vi "CODMn启动命令 (子VI).vi"(10 "CODMn量程切换":enum32{"H", "L", "AUTO"}(ring)=enum."AUTO", 11 "启动测量模式":T1) -> ()   [LabVIEW 2016, in "斯坦道CODMn.lvlib"]
uses:
  <vilib>/Plasmionique/MB Master/MB_Master_Serial/MB_Master_Serial.lvclass
  C:/Program Files (x86)/National Instruments/LabVIEW 2016/vi.lib/Plasmionique/MB Master/MB_Master/MB_Master.lvclass
  <vilib>/Plasmionique/MB Master/MB Master.lvlib
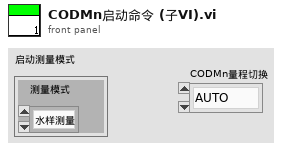
[diagram p1: front panel]
types:
  T1 = cluster{"测量模式":enum16{"水样测量", "标样核查", "零点核查", "跨度核查", "空白测试", "加标回收", "平行样", "校零", "校标"}}
  T2 = cluster{"baud rate (bps)":u32, "stop bits":u16, "parity":u16, "flow control":u16, "timeout":u32, "retries":i32}
  T3 = enum16{"水样测量", "标样核查", "零点核查", "跨度核查", "空白测试", "加标回收", "平行样", "校零", "校标"}
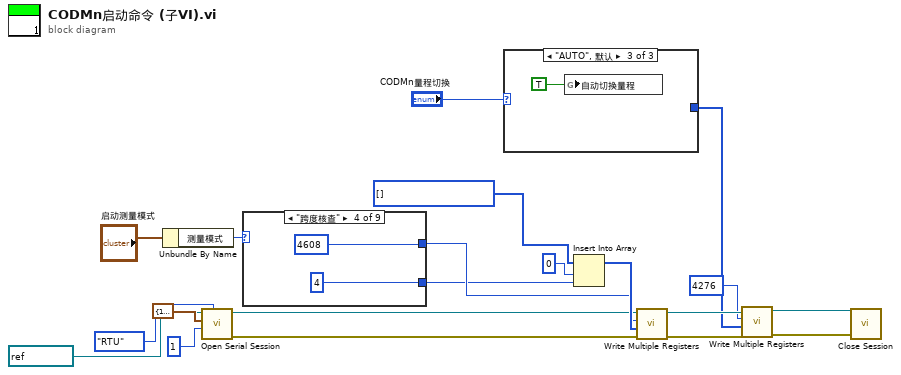
[diagram p0: block diagram]
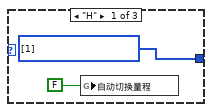
[diagram p2: hidden frame]
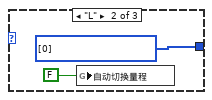
[diagram p3: hidden frame]
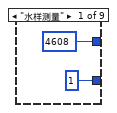
[diagram p4: hidden frame]
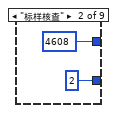
[diagram p5: hidden frame]
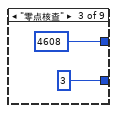
[diagram p6: hidden frame]
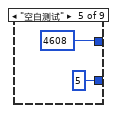
[diagram p7: hidden frame]
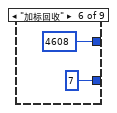
[diagram p8: hidden frame]
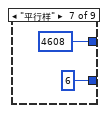
[diagram p9: hidden frame]
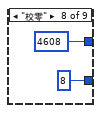
[diagram p10: hidden frame]
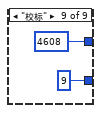
[diagram p11: hidden frame]
diagram:
  n1 = Unbundle By Name("启动测量模式") -> ("测量模式"=w13:T3)
  n2 = call <vilib>:"Open Serial Session.vi"("Mode (RTU)"=enum16{"RTU", "ASCII"}."RTU", "Slave ID"=u8 1, "Serial Config"=T2 {"baud rate (bps)"=115200, "stop bits"=10, "parity"=0, "flow control"=0, "timeout"=1000, "retries"=1}, "VISA Resource"=refnum<visa-resource-name> "COM4") -> ("Error out"=w20:errorcluster, "MB_Serial session"=w8:refnum<class "MB_Master_Serial.lvclass">)  [unwired: 6 in]
  n3 = case shown="\"跨度核查\"" w13 {
    tunnel: [u16 4608 ("address") u16 4608 ("address") u16 4608 ("address") u16 4608 ("address") u16 4608 ("address") u16 4608 ("address") u16 4608 ("address") u16 4608 ("address") u16 4608 ("address")] -> w18
    tunnel: [u16 1 ("address") u16 2 ("address") u16 3 ("address") u16 4 ("address") u16 5 ("address") u16 7 ("address") u16 6 ("address") u16 8 ("address") u16 9 ("address")] -> w11
    frame "水样测量" {
    }
    frame "标样核查" {
    }
    frame "零点核查" {
    }
    frame "跨度核查" {
    }
    frame "空白测试" {
    }
    frame "加标回收" {
    }
    frame "平行样" {
    }
    frame "校零" {
    }
    frame "校标" {
    }
  }
  n4 = case shown="\"AUTO\", 默认" "CODMn量程切换" {
    tunnel: [u16[] [1] ("values") u16[] [0] ("values") _] -> w1
    frame "H" {
      n5 = global write "系统变量.vi" "自动切换量程"(FALSE ("自动切换量程")) -> ()
    }
    frame "L" {
      n6 = global write "系统变量.vi" "自动切换量程"(FALSE ("自动切换量程")) -> ()
    }
    frame "AUTO", Default {
      n7 = global write "系统变量.vi" "自动切换量程"(TRUE ("自动切换量程")) -> ()
    }
  }
  n8 = Insert Into Array(array=u16[] [] ("values"), index=0 ("索引"), new element=w11) -> (w19:u16[])
  n9 = call <vilib>:"Write Multiple Registers.vi"("error in (no error)"=w20, "values"=w19, "starting address"=w18, "MB session in"=w8) -> ("error out"=w6:errorcluster, "MB session out"=w7:refnum<class "MB_Master_Serial.lvclass">)  [unwired: 6 in]
  n10 = call <vilib>:"Write Multiple Registers.vi"("error in (no error)"=w6, "values"=w1, "starting address"=u16 4276, "MB session in"=w7) -> ("error out"=w4:errorcluster, "MB session out"=w5:refnum<class "MB_Master_Serial.lvclass">)  [unwired: 6 in]
  n11 = call-dynamic "Close Session.vi"("error in (no error)"=w4, "MB_Serial session"=w5) -> ()  [unwired: 9 in, 1 out]
